vi "Activation.vi"() -> ()   [LabVIEW 2018]
panel:
  out "提示符":string
  in  "激活":bool
  in  "激活码":string
  out "MAC地址":string
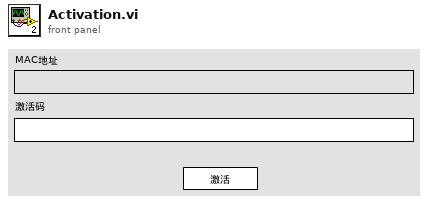
[diagram p1: front panel]
types:
  T1 = cluster{"提示符":refnum<vi>, "激活码":refnum<vi>, "MAC码":refnum<vi>, "激活按钮":refnum<vi>}
  T2 = enum32{"Invalid", "Standard", "Closed", "Hidden", "Minimized", "Maximized"}
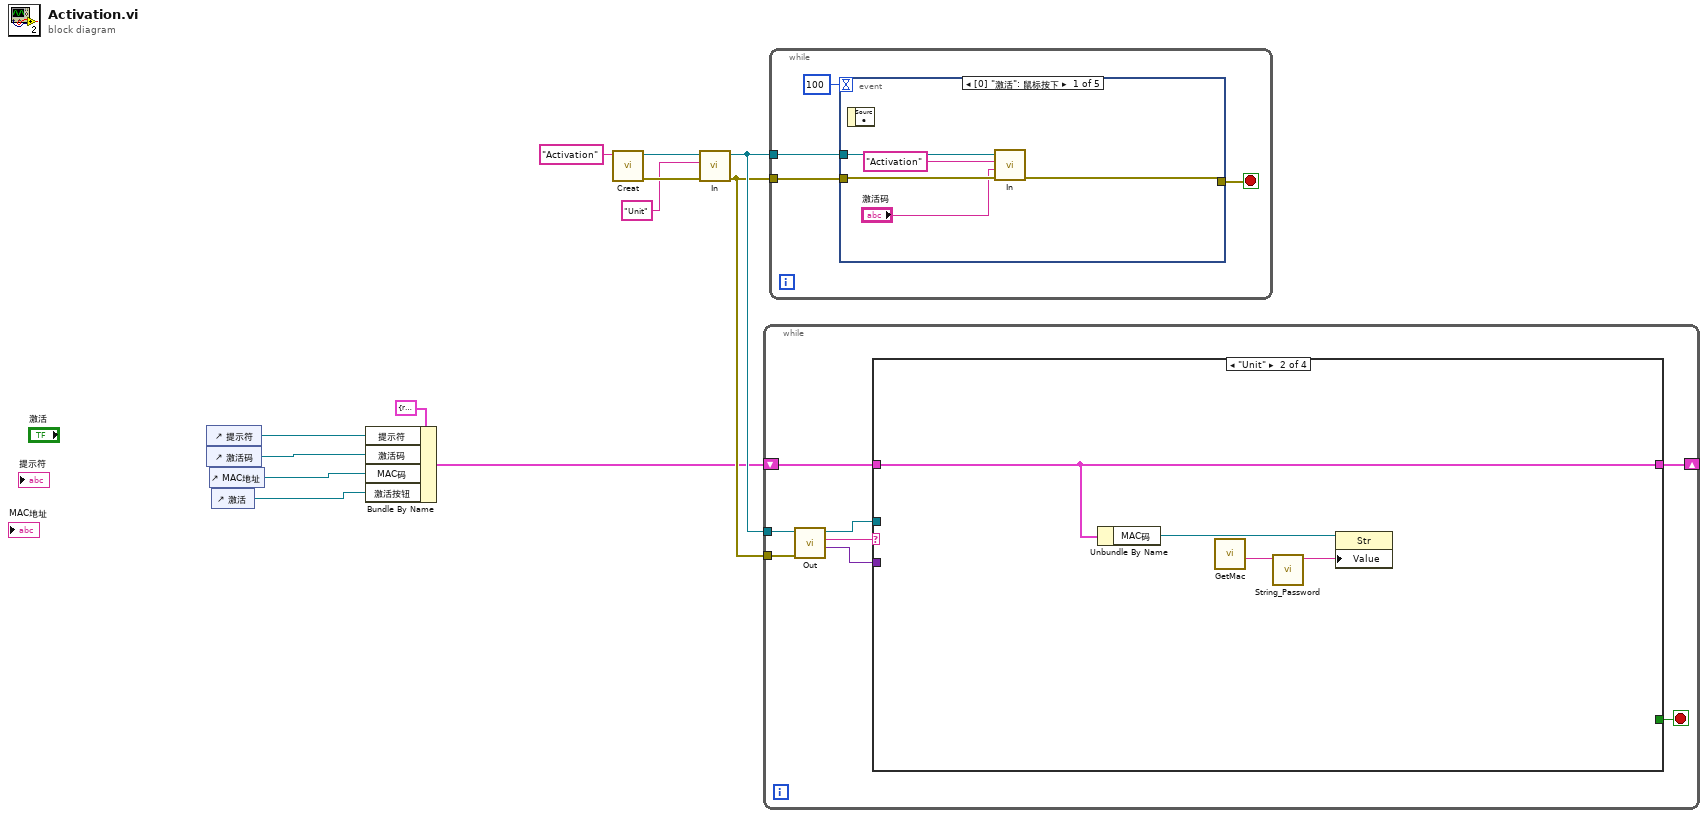
[diagram p0: block diagram]
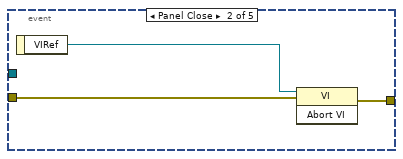
[diagram p2: hidden frame]
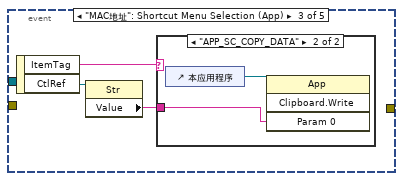
[diagram p3: hidden frame]
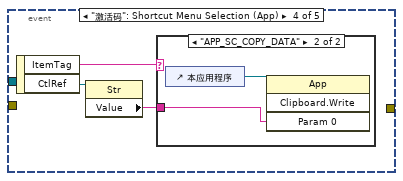
[diagram p5: hidden frame]
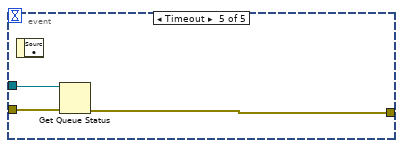
[diagram p7: hidden frame]
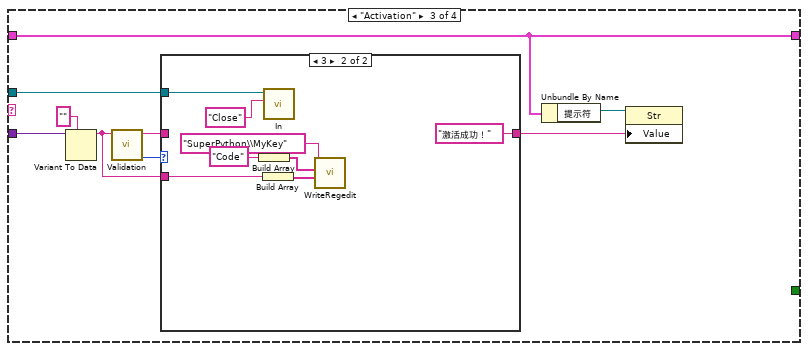
[diagram p9: hidden frame]
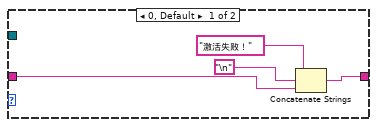
[diagram p10: hidden frame]
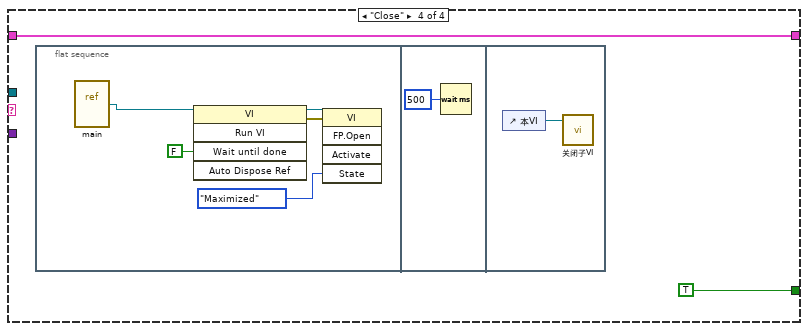
[diagram p11: hidden frame]
diagram:
  n1 = control-ref of="提示符"() -> (w3:refnum<vi>)
  n2 = control-ref of="激活码"() -> (w4:refnum<vi>)
  n3 = control-ref of="MAC地址"() -> (w5:refnum<vi>)
  n4 = control-ref of="激活"() -> (w6:refnum<vi>)
  n5 = Bundle By Name(cluster=T1 {"提示符"=refnum, "激活码"=refnum, "MAC码"=refnum, "激活按钮"=refnum}, "提示符"=w3, "激活码"=w4, "MAC码"=w5, "激活按钮"=w6) -> (w1:T1)
  n6 = call "Creat.vi"("名称"="Activation" ("QueueName")) -> ("错误输出"=w10:errorcluster, "队列输出"=w11:refnum<queue>)  [unwired: 9 in]
  n7 = call "In.vi"("错误输入"=w10, "指令"="Unit" ("Event"), "队列"=w11) -> ("错误输出"=w7:errorcluster, "队列输出"=w8:refnum<queue>)  [unwired: 7 in]
  n8 = while {
    tunnel: w8 -> [w20]
    tunnel: w7 -> [w19]
    shift-right: [w15] -> _
    shift-left: w1 -> [w16]
    stop <- w13 stop-if-true
    n9 = call "Out.vi"("错误输入"=w19, "队列"=w20) -> ("数据"=w17:variant, "指令"=w18:string, "队列输出"=w14:refnum<queue>)  [unwired: 6 in, 1 out]
    n10 = case shown="\"Unit\"" w18 {
      tunnel: w17 -> [_ _ w34 _]
      tunnel: [w21 w25 w29 w48] -> w15
      tunnel: w16 -> [w21 w25 w29 w48]
      tunnel: w14 -> [_ _ w30 _]
      tunnel: [_ _ _ TRUE] -> w13
      frame "NULL", Default {
      }
      frame "Unit" {
        n11 = Unbundle By Name(w25) -> ("MAC码"=w24:refnum<vi>)
        n12 = call "GetMac.vi"() -> ("网络适配器:MAC地址"=w23:string)  [unwired: 10 in, 1 out]
        n13 = call "String_Password.vi"("String"=w23) -> ("Password"=w22:string)  [unwired: 10 in]
        n14 = property class="Str"(reference=w24, "Value"=w22) -> ()  [unwired: 1 in, 2 out]
      }
      frame "Activation" {
        n15 = Variant To Data(type="", Variant=w34) -> (data=w31:string)  [unwired: 1 in, 1 out]
        n16 = call "Validation.vi"("Password"=w31) -> ("激活状态"=w32:i32, "提示符"=w26:string)  [unwired: 8 in, 1 out]
        n17 = case shown="3" w32 {
          tunnel: w31 -> [_ w42]
          tunnel: w30 -> [_ w45]
          tunnel: [w36 "激活成功！" ("提示符")] -> w27
          tunnel: w26 -> [w37 _]
          frame 0, Default {
            n18 = Concatenate Strings("激活失败！" ("提示符"), "\n", w37) -> (w36:string)
          }
          frame 3 {
            n19 = Build Array("Code" ("value")) -> (w41:string[])
            n20 = Build Array(w42) -> (w40:string[])
            n21 = call "In.vi"("指令"="Close" ("Event"), "队列"=w45) -> ()  [unwired: 8 in, 2 out]
            n22 = call "WriteRegedit.vi"("值"=w40, "名称"=w41, "subkey"="SuperPython\\MyKey") -> ()  [unwired: 8 in, 1 out]
          }
        }
        n23 = Unbundle By Name(w29) -> ("提示符"=w28:refnum<vi>)
        n24 = property class="Str"(reference=w28, "Value"=w27) -> ()  [unwired: 1 in, 2 out]
      }
      frame "Close" {
        n25 = flat-sequence {
          frame #0 {
            n26 = vi-ref "main.vi"() -> (w49:refnum<vi>)
            n27 = invoke class="VI" method="Run VI"(reference=w49, "Wait until done"=FALSE ("结束前等待")) -> (reference out=w52:refnum<vi>, error out=w53:errorcluster)  [unwired: 3 in, 3 out]
            n28 = invoke class="VI" method="FP.Open"(reference=w52, error in=w53, "State"=T2."Maximized" ("状态")) -> ()  [unwired: 2 in, 5 out]
          }
          frame #1 {
            n29 = Wait (ms)(milliseconds to wait=u32 500 ("等待时间（毫秒）")) -> ()  [unwired: 1 out]
          }
          frame #2 {
            n30 = control-ref of="本VI"() -> (w55:refnum<vi>)
            n31 = call "关闭子VI.vi"("引用"=w55) -> ()  [unwired: 9 in, 2 out]
          }
        }
      }
    }
  }
  n32 = while {
    tunnel: w8 -> [w59]
    tunnel: w7 -> [w58]
    stop <- w56 stop-if-true
    n33 = event shown="[0] \"激活\": 鼠标按下" {
      selector: _ -> [_ _ _ _ _]
      dyn-events: _ -> [_ _ _ _ _]
      timeout: 100 -> [_ _ _ _ _]
      tunnel: w59 -> [w64 _ _ _ w80]
      tunnel: w58 -> [w63 w65 _ _ w79]
      tunnel: [w60 w66 _ _ w78] -> w56
      event "激活": Mouse Down {
        n34 = event-data() -> ()  [unwired: 1 in, 1 out]
        n35 = call "In.vi"("错误输入"=w63, "数据"="激活码", "指令"="Activation" ("Event"), "队列"=w64) -> ("错误输出"=w60:errorcluster)  [unwired: 6 in, 1 out]
      }
      event Panel Close {
        n36 = event-data() -> ("VIRef"=w67:refnum<vi>)  [unwired: 1 in]
        n37 = invoke class="VI" method="Abort VI"(reference=w67, error in=w65) -> (error out=w66:errorcluster)  [unwired: 1 in, 2 out]
      }
      event "MAC地址": Shortcut Menu Selection (App) {
        n38 = event-data() -> ("ItemTag"=w69:string, "CtlRef"=w70:refnum<vi>)  [unwired: 1 in]
        n39 = property class="Str"(reference=w70) -> ("Value"=w68:string)  [unwired: 1 in, 2 out]
        n40 = case shown="\"APP_SC_COPY_DATA\"" w69 {
          tunnel: w68 -> [_ w71]
          frame "假", Default {
          }
          frame "APP_SC_COPY_DATA" {
            n41 = control-ref of="本应用程序"() -> (w72:refnum<vi>)
            n42 = invoke class="App" method="Clipboard.Write"(reference=w72, "Param 0"=w71) -> ()  [unwired: 2 in, 4 out]
          }
        }
      }
      event "激活码": Shortcut Menu Selection (App) {
        n43 = event-data() -> ("ItemTag"=w74:string, "CtlRef"=w75:refnum<vi>)  [unwired: 1 in]
        n44 = property class="Str"(reference=w75) -> ("Value"=w73:string)  [unwired: 1 in, 2 out]
        n45 = case shown="\"APP_SC_COPY_DATA\"" w74 {
          tunnel: w73 -> [_ w76]
          frame "假", Default {
          }
          frame "APP_SC_COPY_DATA" {
            n46 = control-ref of="本应用程序"() -> (w77:refnum<vi>)
            n47 = invoke class="App" method="Clipboard.Write"(reference=w77, "Param 0"=w76) -> ()  [unwired: 2 in, 4 out]
          }
        }
      }
      event Timeout {
        n48 = event-data() -> ()  [unwired: 1 in, 1 out]
        n49 = Get Queue Status(queue=w80, error in (no error)=w79) -> (error out=w78:errorcluster)  [unwired: 1 in, 7 out]
      }
    }
  }
